vi "App Parameters Dialog.vi"(8 "error in (no error)":errorcluster) -> (0 "error out":errorcluster)   [LabVIEW 2013]
uses:
  lib/Data Access Objects/Application/Timing & Logging Parameters.ctl
  lib/Data Access Objects/Application/Timing Parameters.ctl
  lib/Apps/App Parameters Actions.ctl
  lib/Logging/Log Filename Actions.ctl
panel:
  in  "OK":bool
  in  "Application Timing and Logging":T1
  # "Interval is in Seconds\nRate is in Samples per Second"
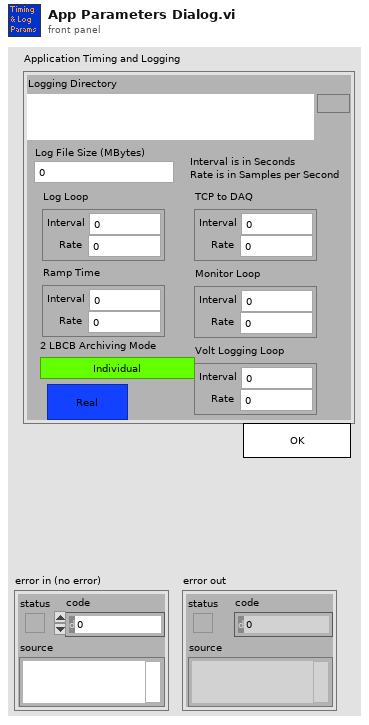
[diagram p1: front panel]
types:
  T1 = typedef "Timing & Logging Parameters.ctl" = cluster{"Monitor Loop":T2, "Ramp Time":T2, "Log Loop":T2, "TCP to DAQ":T2, "Logging Directory":path, "Log File Size (MBytes)":i64, "Volt Logging Loop":T2, "2 LBCB Archiving Mode":bool, "Fake":bool}
  T2 = typedef "Timing Parameters.ctl" = cluster{"Interval":dbl, "Rate ":dbl}
  T3 = typedef "App Parameters Actions.ctl" = enum16{"Init", "Get", "Set"}
  T4 = typedef "Log Filename Actions.ctl" = enum16{"Init", "Get Filename", "New Log Directory"}
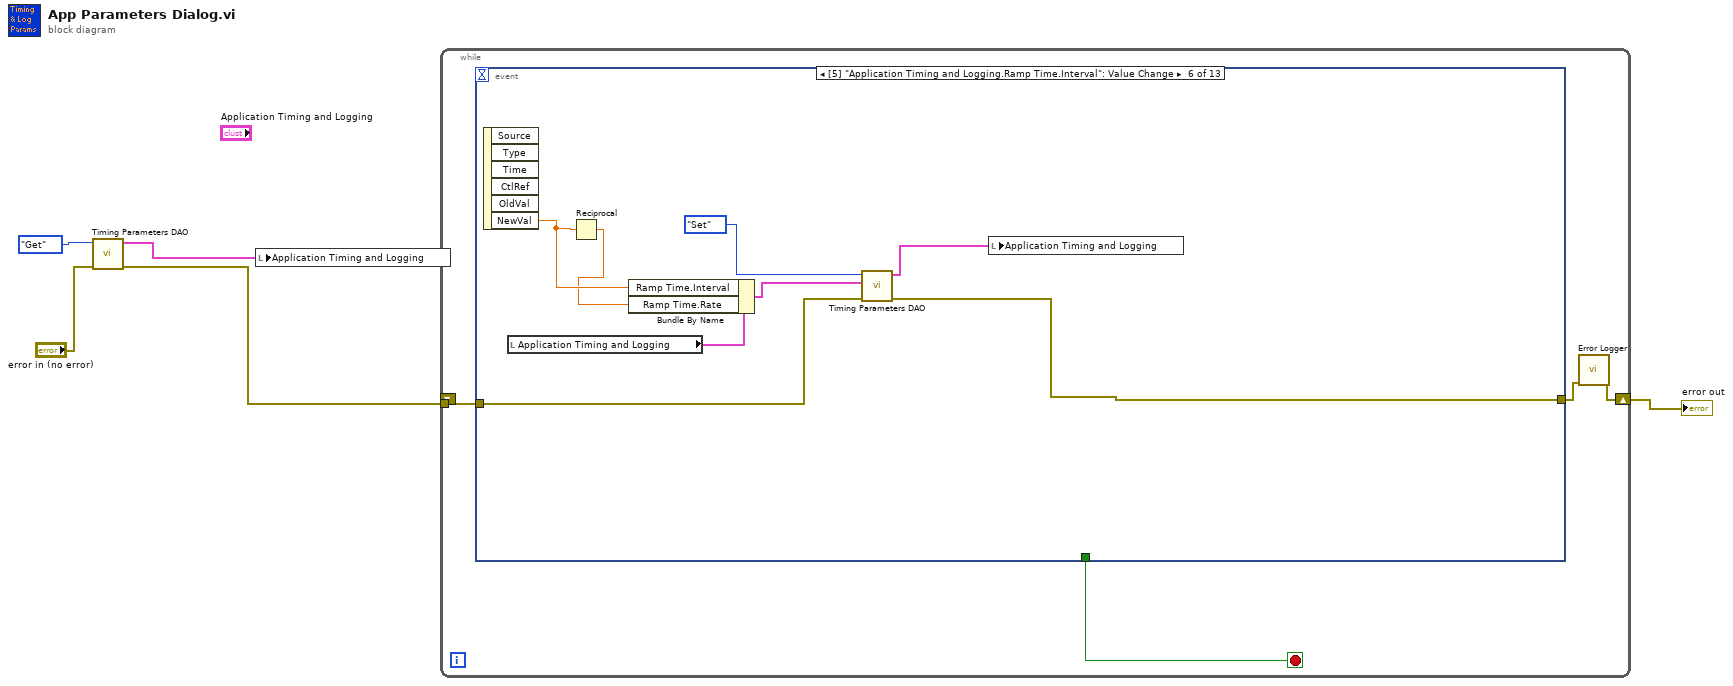
[diagram p0: block diagram]
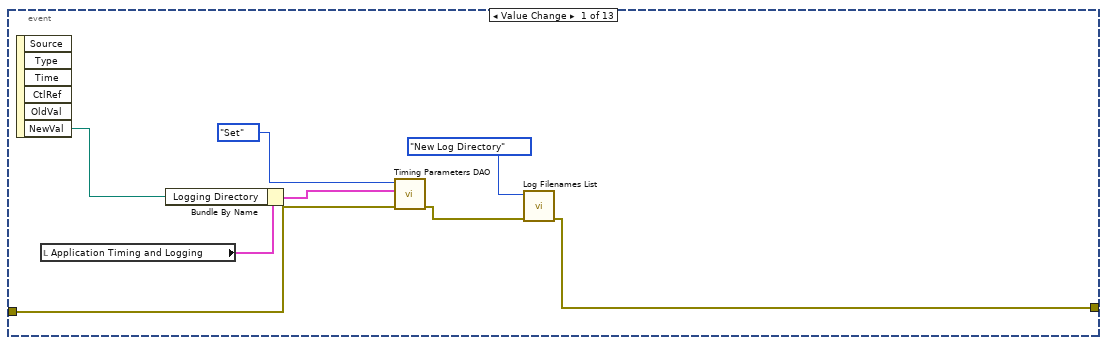
[diagram p2: hidden frame]
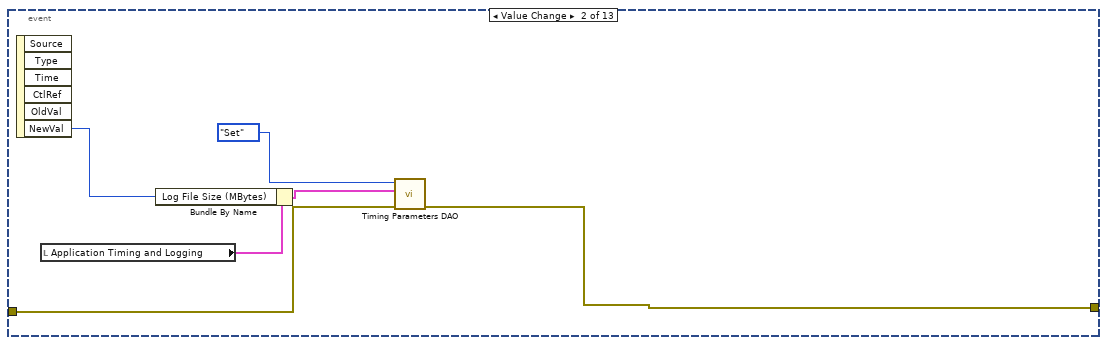
[diagram p3: hidden frame]
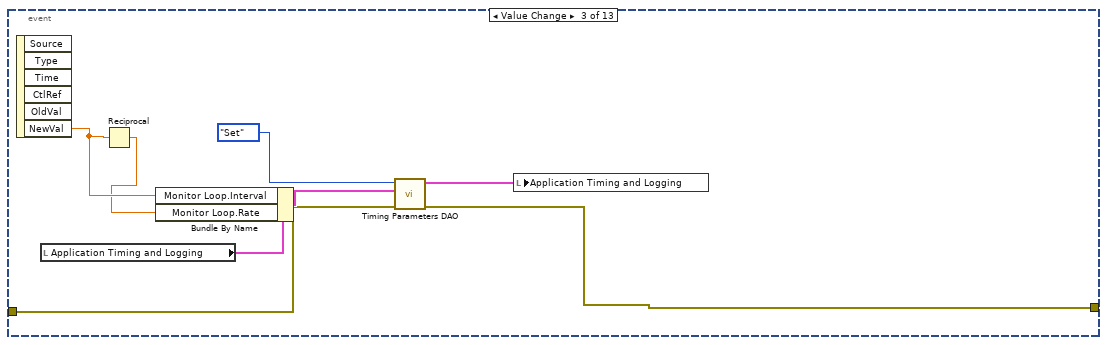
[diagram p4: hidden frame]
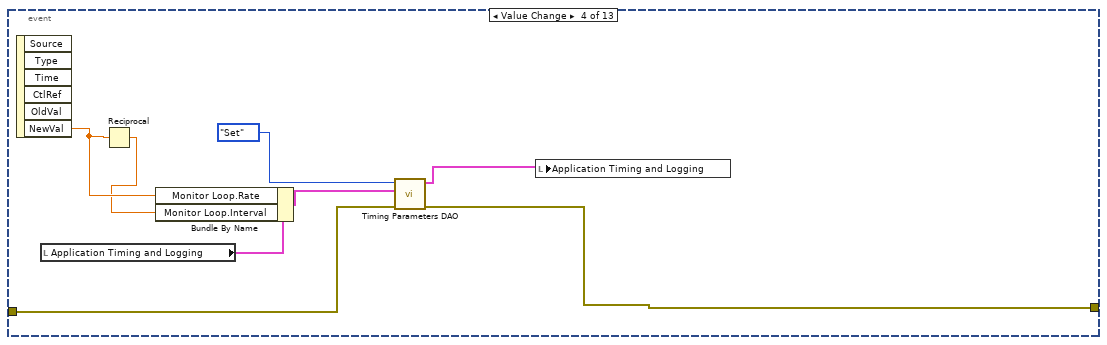
[diagram p5: hidden frame]
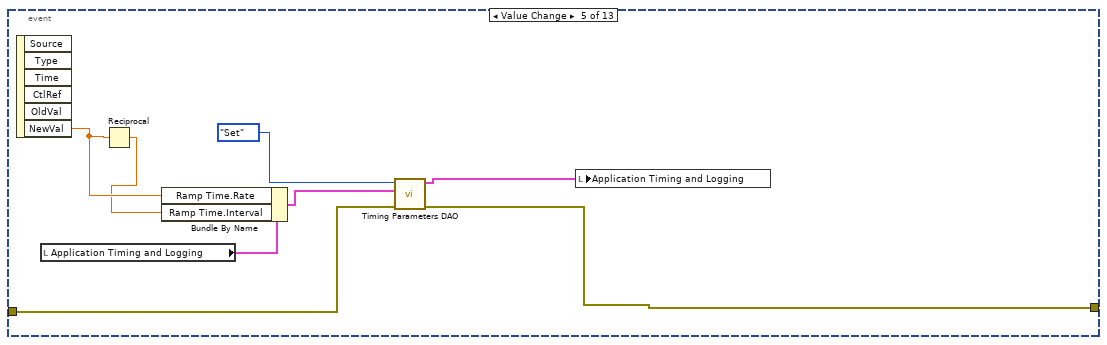
[diagram p6: hidden frame]
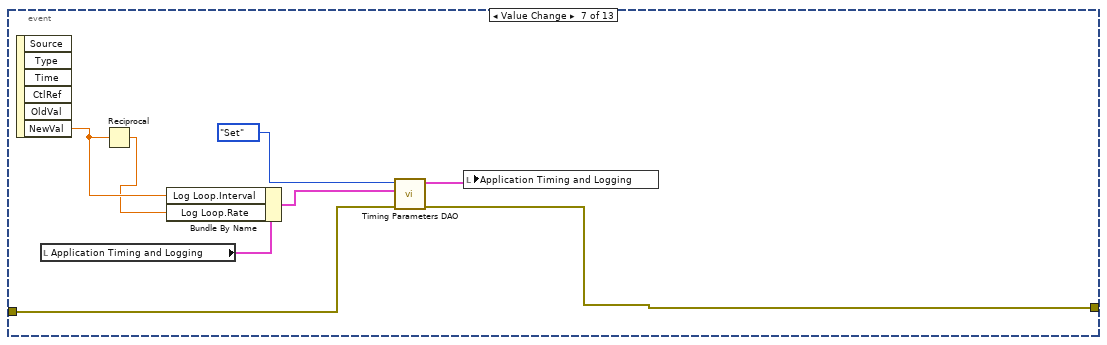
[diagram p7: hidden frame]
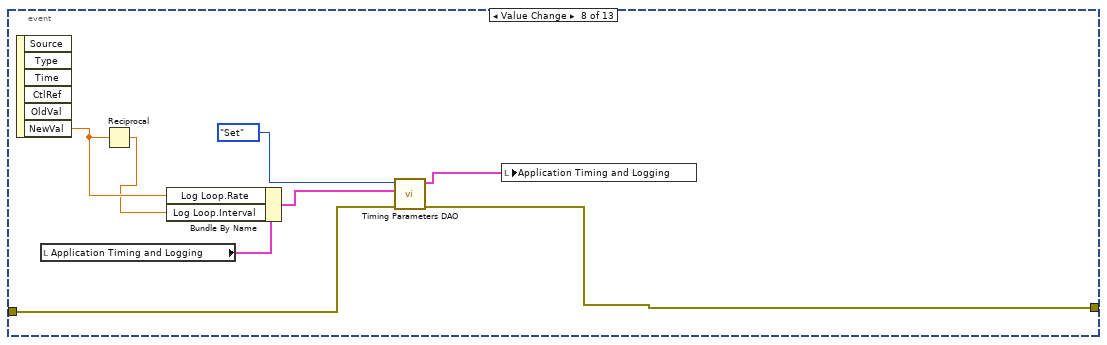
[diagram p8: hidden frame]
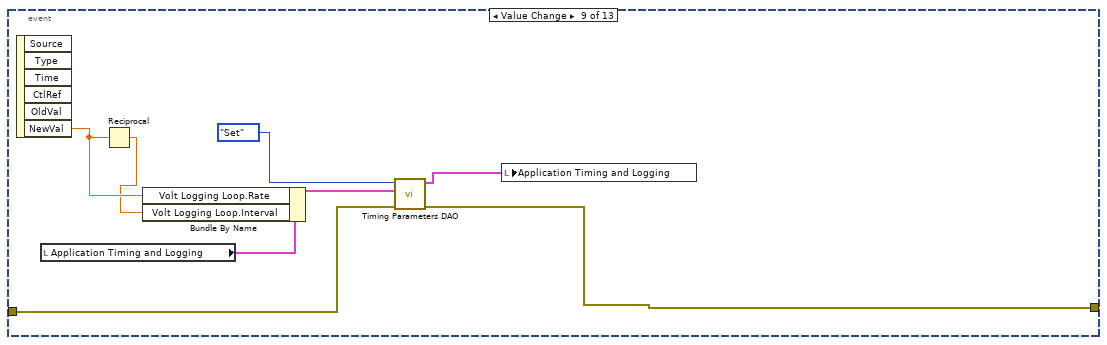
[diagram p9: hidden frame]
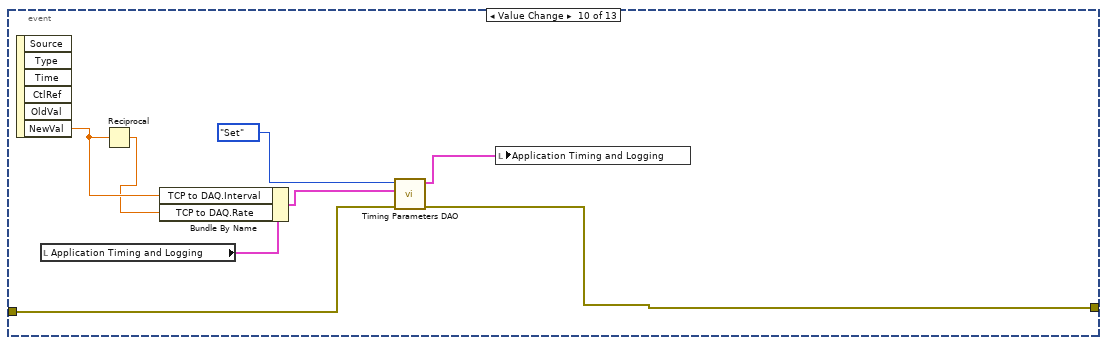
[diagram p10: hidden frame]
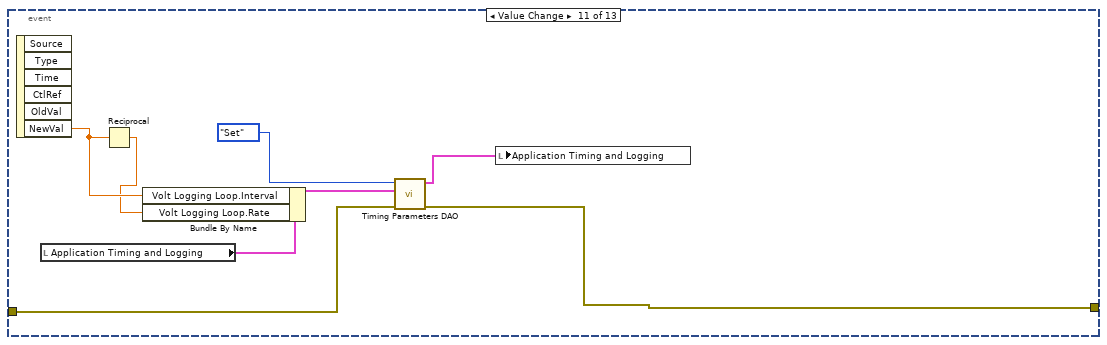
[diagram p11: hidden frame]
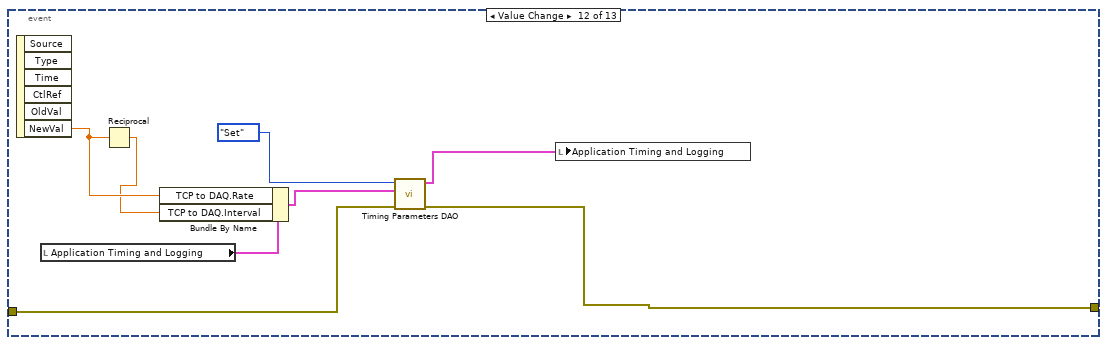
[diagram p12: hidden frame]
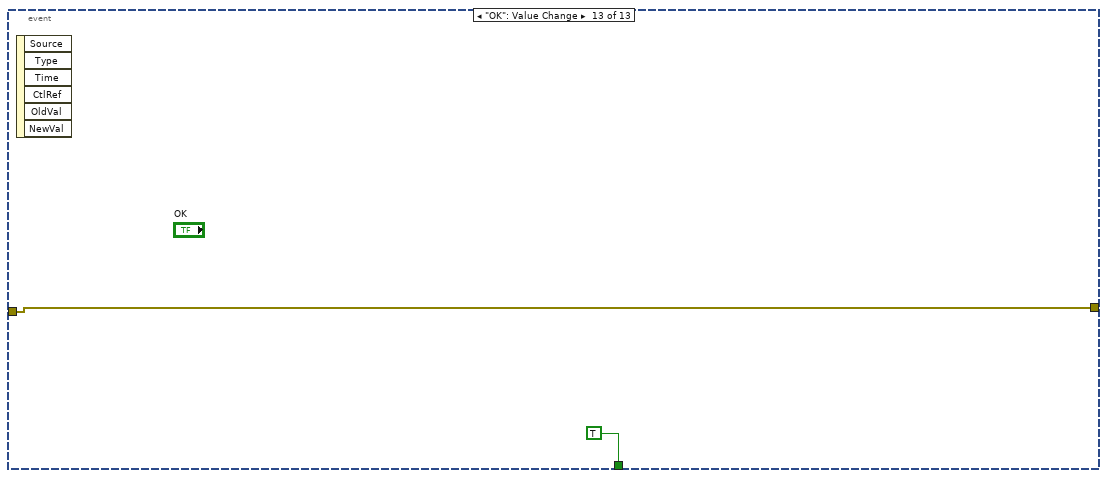
[diagram p13: hidden frame]
diagram:
  n1 = call "Timing Parameters DAO.vi"("error in (no error)"="error in (no error)", "Actions"=App_Parameters_Actions."Get" ("App Parameter Actions")) -> ("error out"=w1:errorcluster, "Application Timing and Logging Out"=w4:T1)  [unwired: 2 in, 6 out]
  n2 = local write "Application Timing and Logging"(w4) -> ()
  n3 = while {
    tunnel: w1 -> [w9]
    shift-right: [w6] -> w3
    shift-left: _ -> [_]
    stop <- w8 stop-if-true
    n4 = event shown="[5] \"Application Timing and Logging.Ramp Time.Interval\": Value Change" {
      selector: _ -> [_ _ _ _ _ _ _ _ _ _ _ _ _]
      dyn-events: _ -> [_ _ _ _ _ _ _ _ _ _ _ _ _]
      timeout: _ -> [_ _ _ _ _ _ _ _ _ _ _ _ _]
      tunnel: w9 -> [w13 w19 w28 w36 w44 w52 w60 w68 w76 w84 w92 w100 w104]
      tunnel: [w10 w18 w27 w35 w43 w51 w59 w67 w75 w83 w91 w99 w104] -> w7
      tunnel: [_ _ _ _ _ _ _ _ _ _ _ _ TRUE] -> w8
      event Value Change {
        n5 = event-data() -> ("NewVal"=w14:path)  [unwired: 6 out]
        n6 = local read "Application Timing and Logging"() -> (w17:T1)
        n7 = Bundle By Name(cluster=w17, "Logging Directory"=w14) -> (w15:T1)
        n8 = call "Timing Parameters DAO.vi"("error in (no error)"=w13, "Application Timing and Logging In"=w15, "Actions"=App_Parameters_Actions."Set" ("App Parameter Actions")) -> ("error out"=w12:errorcluster)  [unwired: 1 in, 7 out]
        n9 = call "Log Filenames List.vi"("error in (no error)"=w12, "Log Filename Actions"=Log_Filename_Actions."New Log Directory") -> ("error out"=w10:errorcluster)  [unwired: 2 in, 7 out]
      }
      event Value Change {
        n10 = event-data() -> ("NewVal"=w20:i64)  [unwired: 6 out]
        n11 = local read "Application Timing and Logging"() -> (w23:T1)
        n12 = Bundle By Name(cluster=w23, "Log File Size (MBytes)"=w20) -> (w21:T1)
        n13 = call "Timing Parameters DAO.vi"("error in (no error)"=w19, "Application Timing and Logging In"=w21, "Actions"=App_Parameters_Actions."Set" ("App Parameter Actions")) -> ("error out"=w18:errorcluster)  [unwired: 1 in, 7 out]
      }
      event Value Change {
        n14 = event-data() -> ("NewVal"=w26:dbl)  [unwired: 6 out]
        n15 = local read "Application Timing and Logging"() -> (w31:T1)
        n16 = Reciprocal(x=w26) -> (1/x=w25:dbl)
        n17 = Bundle By Name(cluster=w31, "Monitor Loop.Interval"=w26, "Monitor Loop.Rate"=w25) -> (w29:T1)
        n18 = call "Timing Parameters DAO.vi"("error in (no error)"=w28, "Application Timing and Logging In"=w29, "Actions"=App_Parameters_Actions."Set" ("App Parameter Actions")) -> ("error out"=w27:errorcluster, "Application Timing and Logging Out"=w24:T1)  [unwired: 1 in, 6 out]
        n19 = local write "Application Timing and Logging"(w24) -> ()
      }
      event Value Change {
        n20 = event-data() -> ("NewVal"=w34:dbl)  [unwired: 6 out]
        n21 = local read "Application Timing and Logging"() -> (w39:T1)
        n22 = Reciprocal(x=w34) -> (1/x=w33:dbl)
        n23 = Bundle By Name(cluster=w39, "Monitor Loop.Rate"=w34, "Monitor Loop.Interval"=w33) -> (w37:T1)
        n24 = call "Timing Parameters DAO.vi"("error in (no error)"=w36, "Application Timing and Logging In"=w37, "Actions"=App_Parameters_Actions."Set" ("App Parameter Actions")) -> ("error out"=w35:errorcluster, "Application Timing and Logging Out"=w32:T1)  [unwired: 1 in, 6 out]
        n25 = local write "Application Timing and Logging"(w32) -> ()
      }
      event Value Change {
        n26 = event-data() -> ("NewVal"=w42:dbl)  [unwired: 6 out]
        n27 = local read "Application Timing and Logging"() -> (w47:T1)
        n28 = Reciprocal(x=w42) -> (1/x=w41:dbl)
        n29 = Bundle By Name(cluster=w47, "Ramp Time.Rate"=w42, "Ramp Time.Interval"=w41) -> (w45:T1)
        n30 = call "Timing Parameters DAO.vi"("error in (no error)"=w44, "Application Timing and Logging In"=w45, "Actions"=App_Parameters_Actions."Set" ("App Parameter Actions")) -> ("error out"=w43:errorcluster, "Application Timing and Logging Out"=w40:T1)  [unwired: 1 in, 6 out]
        n31 = local write "Application Timing and Logging"(w40) -> ()
      }
      event Value Change {
        n32 = event-data() -> ("NewVal"=w50:dbl)  [unwired: 6 out]
        n33 = local read "Application Timing and Logging"() -> (w55:T1)
        n34 = Reciprocal(x=w50) -> (1/x=w49:dbl)
        n35 = Bundle By Name(cluster=w55, "Ramp Time.Interval"=w50, "Ramp Time.Rate"=w49) -> (w53:T1)
        n36 = call "Timing Parameters DAO.vi"("error in (no error)"=w52, "Application Timing and Logging In"=w53, "Actions"=App_Parameters_Actions."Set" ("App Parameter Actions")) -> ("error out"=w51:errorcluster, "Application Timing and Logging Out"=w48:T1)  [unwired: 1 in, 6 out]
        n37 = local write "Application Timing and Logging"(w48) -> ()
      }
      event Value Change {
        n38 = event-data() -> ("NewVal"=w58:dbl)  [unwired: 6 out]
        n39 = local read "Application Timing and Logging"() -> (w63:T1)
        n40 = Reciprocal(x=w58) -> (1/x=w57:dbl)
        n41 = Bundle By Name(cluster=w63, "Log Loop.Interval"=w58, "Log Loop.Rate"=w57) -> (w61:T1)
        n42 = call "Timing Parameters DAO.vi"("error in (no error)"=w60, "Application Timing and Logging In"=w61, "Actions"=App_Parameters_Actions."Set" ("App Parameter Actions")) -> ("error out"=w59:errorcluster, "Application Timing and Logging Out"=w56:T1)  [unwired: 1 in, 6 out]
        n43 = local write "Application Timing and Logging"(w56) -> ()
      }
      event Value Change {
        n44 = event-data() -> ("NewVal"=w66:dbl)  [unwired: 6 out]
        n45 = local read "Application Timing and Logging"() -> (w71:T1)
        n46 = Reciprocal(x=w66) -> (1/x=w65:dbl)
        n47 = Bundle By Name(cluster=w71, "Log Loop.Rate"=w66, "Log Loop.Interval"=w65) -> (w69:T1)
        n48 = call "Timing Parameters DAO.vi"("error in (no error)"=w68, "Application Timing and Logging In"=w69, "Actions"=App_Parameters_Actions."Set" ("App Parameter Actions")) -> ("error out"=w67:errorcluster, "Application Timing and Logging Out"=w64:T1)  [unwired: 1 in, 6 out]
        n49 = local write "Application Timing and Logging"(w64) -> ()
      }
      event Value Change {
        n50 = event-data() -> ("NewVal"=w74:dbl)  [unwired: 6 out]
        n51 = local read "Application Timing and Logging"() -> (w79:T1)
        n52 = Reciprocal(x=w74) -> (1/x=w73:dbl)
        n53 = Bundle By Name(cluster=w79, "Volt Logging Loop.Rate"=w74, "Volt Logging Loop.Interval"=w73) -> (w77:T1)
        n54 = call "Timing Parameters DAO.vi"("error in (no error)"=w76, "Application Timing and Logging In"=w77, "Actions"=App_Parameters_Actions."Set" ("App Parameter Actions")) -> ("error out"=w75:errorcluster, "Application Timing and Logging Out"=w72:T1)  [unwired: 1 in, 6 out]
        n55 = local write "Application Timing and Logging"(w72) -> ()
      }
      event Value Change {
        n56 = event-data() -> ("NewVal"=w82:dbl)  [unwired: 6 out]
        n57 = local read "Application Timing and Logging"() -> (w87:T1)
        n58 = Reciprocal(x=w82) -> (1/x=w81:dbl)
        n59 = Bundle By Name(cluster=w87, "TCP to DAQ.Interval"=w82, "TCP to DAQ.Rate"=w81) -> (w85:T1)
        n60 = call "Timing Parameters DAO.vi"("error in (no error)"=w84, "Application Timing and Logging In"=w85, "Actions"=App_Parameters_Actions."Set" ("App Parameter Actions")) -> ("error out"=w83:errorcluster, "Application Timing and Logging Out"=w80:T1)  [unwired: 1 in, 6 out]
        n61 = local write "Application Timing and Logging"(w80) -> ()
      }
      event Value Change {
        n62 = event-data() -> ("NewVal"=w90:dbl)  [unwired: 6 out]
        n63 = local read "Application Timing and Logging"() -> (w95:T1)
        n64 = Reciprocal(x=w90) -> (1/x=w89:dbl)
        n65 = Bundle By Name(cluster=w95, "Volt Logging Loop.Interval"=w90, "Volt Logging Loop.Rate"=w89) -> (w93:T1)
        n66 = call "Timing Parameters DAO.vi"("error in (no error)"=w92, "Application Timing and Logging In"=w93, "Actions"=App_Parameters_Actions."Set" ("App Parameter Actions")) -> ("error out"=w91:errorcluster, "Application Timing and Logging Out"=w88:T1)  [unwired: 1 in, 6 out]
        n67 = local write "Application Timing and Logging"(w88) -> ()
      }
      event Value Change {
        n68 = event-data() -> ("NewVal"=w98:dbl)  [unwired: 6 out]
        n69 = local read "Application Timing and Logging"() -> (w103:T1)
        n70 = Reciprocal(x=w98) -> (1/x=w97:dbl)
        n71 = Bundle By Name(cluster=w103, "TCP to DAQ.Rate"=w98, "TCP to DAQ.Interval"=w97) -> (w101:T1)
        n72 = call "Timing Parameters DAO.vi"("error in (no error)"=w100, "Application Timing and Logging In"=w101, "Actions"=App_Parameters_Actions."Set" ("App Parameter Actions")) -> ("error out"=w99:errorcluster, "Application Timing and Logging Out"=w96:T1)  [unwired: 1 in, 6 out]
        n73 = local write "Application Timing and Logging"(w96) -> ()
      }
      event "OK": Value Change {
        n74 = event-data() -> ()  [unwired: 7 out]
      }
    }
    n75 = call "Error Logger.vi"("error in (no error)"=w7) -> ("error out"=w6:errorcluster)  [unwired: 1 in, 9 out]
  }
  "error out" <- w3
